vi "WriteTree.vi"(8 "error in":errorcluster, 11 "CEF_Repository in":refnum<class "CEF_Repository.lvclass">) -> (0 "error out":errorcluster, 2 "root":T1, 3 "CEF_Repository out":refnum<class "CEF_Repository.lvclass">)   [LabVIEW 2025, in "CEF.lvlib" / "CEF_Repository.lvclass"]
doc: "Transfers information between the repo and the tree control. This method should be called after the custom views are called or saving to disk.Copyright 2017 National Instruments Corporation\n\nLicensed under the Apache License, Version 2.0 (the \"License\"); you may not use this file except in compliance with the License. You may obtain a copy of the License at http://www.apache.org/licenses/LICENSE-2.0\nUnless required by applicable law or agreed to in writing, software distributed under the License is distributed on an \"AS IS\" BASIS, WITHOUT WARRANTIES OR CONDITIONS OF ANY KIND, either express or implied. See the License for the specific language governing permissions and limitations under the License."
uses:
  CEF_Repository.lvclass
  Node/NodeRef.ctl
  Node/CEF_Node.lvclass
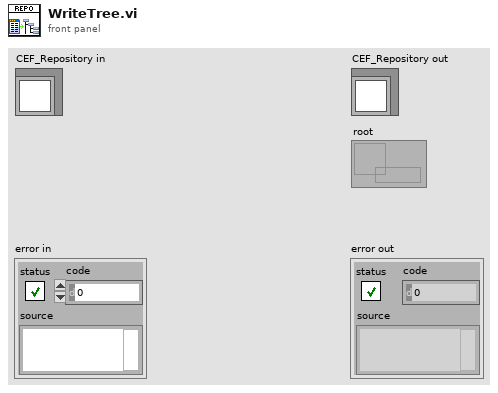
[diagram p1: front panel]
types:
  T1 = typedef "CEF.lvlib/CEF_Node.lvclass/NodeRef.ctl" = refnum<data-value>
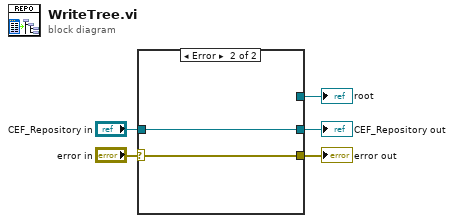
[diagram p0: block diagram]
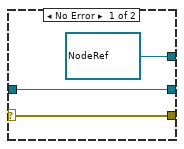
[diagram p2: hidden frame]
diagram:
  n1 = case shown="Error" "error in" {
    selector: "error in" -> [w7 w10]
    tunnel: [w7 w10] -> w4
    tunnel: [w8 w9] -> w2
    tunnel: "CEF_Repository in" -> [w8 w9]
    tunnel: [T1 refnum ("root") _] -> w1
    frame No Error {
    }
    frame Error {
    }
  }
  "error out" <- w4
  "CEF_Repository out" <- w2
  "root" <- w1
